vi "Append log.vi"(10 "message":string, 11 "PrintToSingleFileHtml in":refnum<class "PrintToSingleFileHtml.lvclass">) -> (3 "PrintToSingleFileHtml out":refnum<class "PrintToSingleFileHtml.lvclass">)   [LabVIEW 2026, in "PrintToSingleFileHtml.lvclass"]
uses:
  PrintToSingleFileHtml.lvclass
  PrintToSingleFileHtml.lvclass/PrintToSingleFileHtml.ctl
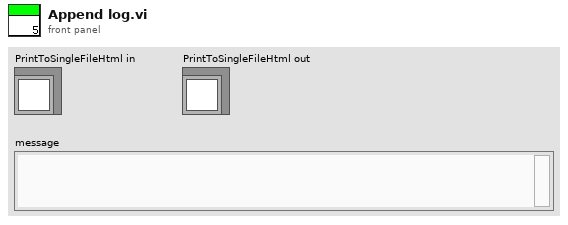
[diagram p1: front panel]
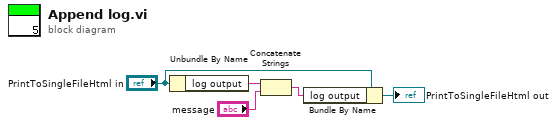
[diagram p0: block diagram]
diagram:
  n1 = Unbundle By Name("PrintToSingleFileHtml in") -> ("log output"=w3:string)
  n2 = Concatenate Strings(w3, "message") -> (w1:string)
  n3 = Bundle By Name(cluster="PrintToSingleFileHtml in", "log output"=w1) -> (→"PrintToSingleFileHtml out":refnum<class "PrintToSingleFileHtml.lvclass">)
